vi "FlatToRichnixnet_grpc_ConvertByteArrayToFramesSinglePointRequest.vi"(5 "OutputClusterType":T1, 11 "InputCluster":T3) -> (3 "OutputCluster":T1)   [LabVIEW 2025, in "xnet-grpc_client.lvlib"]
uses:
  nixnet_grpc_ConvertByteArrayToFramesSinglePointRequest_Flat.ctl
  nidevice_grpc_Session_Flat.ctl
  nixnet_grpc_Protocol.ctl
  nixnet_grpc_ConvertByteArrayToFramesSinglePointRequest.ctl
  nixnet_grpc_ConvertByteArrayToFramesSinglePointRequest_protocol_enum/nixnet_grpc_ConvertByteArrayToFramesSinglePointRequest_protocol_enum.lvclass
  nidevice_grpc_Session.ctl
  xnet-grpc_client.lvlib
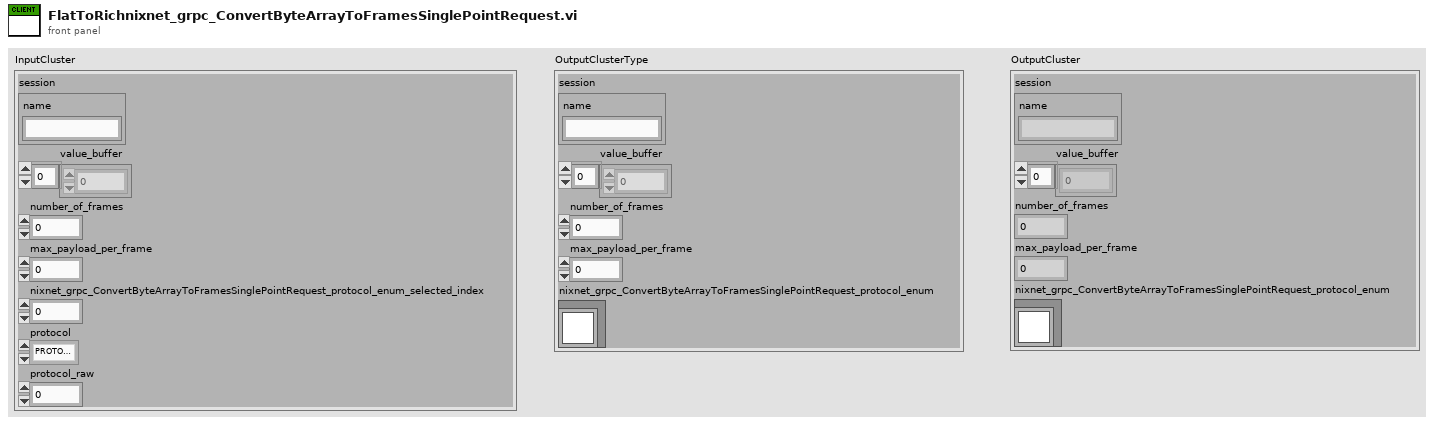
[diagram p1: front panel]
types:
  T1 = typedef "xnet-grpc_client.lvlib/nixnet_grpc_ConvertByteArrayToFramesSinglePointRequest.ctl" = cluster{"session":T2, "value_buffer":u8[], "number_of_frames":u32, "max_payload_per_frame":u32, "nixnet_grpc_ConvertByteArrayToFramesSinglePointRequest_protocol_enum":refnum<class "nixnet_grpc_ConvertByteArrayToFramesSinglePointRequest_protocol_enum.lvclass">}
  T2 = typedef "xnet-grpc_client.lvlib/nidevice_grpc_Session.ctl" = cluster{"name":string}
  T3 = typedef "xnet-grpc_client.lvlib/nixnet_grpc_ConvertByteArrayToFramesSinglePointRequest_Flat.ctl" = cluster{"session":T4, "value_buffer":u8[], "number_of_frames":u32, "max_payload_per_frame":u32, "nixnet_grpc_ConvertByteArrayToFramesSinglePointRequest_protocol_enum_selected_index":i32, "protocol":T5, "protocol_raw":u32}
  T4 = typedef "xnet-grpc_client.lvlib/nidevice_grpc_Session_Flat.ctl" = cluster{"name":string}
  T5 = typedef "xnet-grpc_client.lvlib/nixnet_grpc_Protocol.ctl" = enum32{"PROTOCOL_UNSPECIFIED", "PROTOCOL_CAN", "PROTOCOL_LIN", "PROTOCOL_FLEX_RAY", "PROTOCOL_J1939", "PROTOCOL_ENET"}
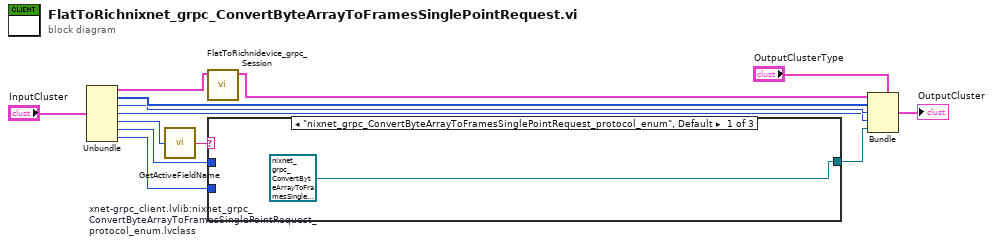
[diagram p0: block diagram]
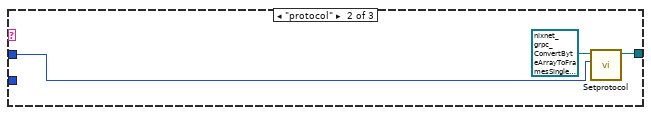
[diagram p2: hidden frame]
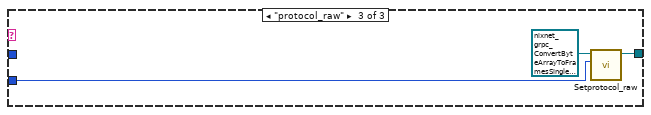
[diagram p3: hidden frame]
diagram:
  n1 = Unbundle "Unbundle"("InputCluster") -> ("session"=w10:T4, "value_buffer"=w8:u8[], "number_of_frames"=w7:u32, "max_payload_per_frame"=w6:u32, "nixnet_grpc_ConvertByteArrayToFramesSinglePointRequest_protocol_enum_selected_index"=w5:i32, "protocol"=w2:T5, "protocol_raw"=w1:u32)
  n2 = call "GetActiveFieldName.vi"("protobuf index"=w5) -> ("oneof field name"=w4:string)
  n3 = call "FlatToRichnidevice_grpc_Session.vi"("InputCluster"=w10) -> ("OutputCluster"=w9:T2)  [unwired: 10 in]
  n4 = case "nixnet_grpc_ConvertByteArrayToFramesSinglePointRequest_protocol_enum" shown="\"nixnet_grpc_ConvertByteArrayToFramesSinglePointRequest_protocol_enum\", Default" w4 {
    tunnel: [w14 w16 w19] -> w3
    tunnel: w2 -> [_ w17 _]
    tunnel: w1 -> [_ _ w20]
    frame "nixnet_grpc_ConvertByteArrayToFramesSinglePointRequest_protocol_enum", Default {
      w14 = refnum<class "nixnet_grpc_ConvertByteArrayToFramesSinglePointRequest_protocol_enum.lvclass"> refnum  # xnet-grpc_client.lvlib:nixnet_grpc_ConvertByteArrayToFramesSinglePointRequest_protocol_enum.lvclass
    }
    frame "protocol" {
      n5 = call "Setprotocol.vi"("Set_Val"=w17, "OneOfTemplate in"=refnum<class "nixnet_grpc_ConvertByteArrayToFramesSinglePointRequest_protocol_enum.lvclass"> refnum) -> ("OneOfTemplate out"=w16:refnum<class "nixnet_grpc_ConvertByteArrayToFramesSinglePointRequest_protocol_enum.lvclass">)  [unwired: 8 in, 1 out]
    }
    frame "protocol_raw" {
      n6 = call "Setprotocol_raw.vi"("Set_Val"=w20, "OneOfTemplate in"=refnum<class "nixnet_grpc_ConvertByteArrayToFramesSinglePointRequest_protocol_enum.lvclass"> refnum) -> ("OneOfTemplate out"=w19:refnum<class "nixnet_grpc_ConvertByteArrayToFramesSinglePointRequest_protocol_enum.lvclass">)  [unwired: 8 in, 1 out]
    }
  }
  n7 = Bundle "Bundle"(cluster="OutputClusterType", "session"=w9, "value_buffer"=w8, "number_of_frames"=w7, "max_payload_per_frame"=w6, "nixnet_grpc_ConvertByteArrayToFramesSinglePointRequest_protocol_enum"=w3) -> (→"OutputCluster":T1)
